vi "RSZVB Set Display Results State.vi"(7 "Display Results (F: Off)":bool, 8 "error in (no error)":errorcluster {"code" format="%.0x"}, 9 "Result Type (0: Phase Delay/El Length)":i32(ring) items=["Phase Delay/El Length", "Min/Max/Peak-Peak", "Mean/Std Dev", "RMS", "Gain/Slope/Flatness", "Compression Point"], 10 "Channel (Trace) (1)":i32=1, 11 "VISA session":refnum<visa-resource-name>) -> (0 "error out":errorcluster {"code" format="%.0x"}, 3 "dup VISA session":refnum<visa-resource-name>)   [LabVIEW 2011]
doc: "This VI displays or hides the Phase Delay/El Length, Min/Max/Peak-Peak, Mean/Std Dev, RMS, Gain/Slope/Flatness or Compression Point results in the diagram area of trace no. <Chn>.\n\nRemote-control command(s):\nCALCulate<Chn>:STATistics:EPDelay[:STATe] <Boolean>\nCALCulate<Chn>:STATistics:MMPTpeak[:STATe] <Boolean>\nCALCulate<Chn>:STATistics:MSTDdev[:STATe] <Boolean>\nCALCulate<Chn>:STATistics:RMS[:STATe] <Boolean>\nCALCulate<Chn>:STATistics:SFLatness[:STATe] <Boolean>\nCALCulate<Chn>:STATistics:NLINear:COMP[:STATe] <Boolean>"
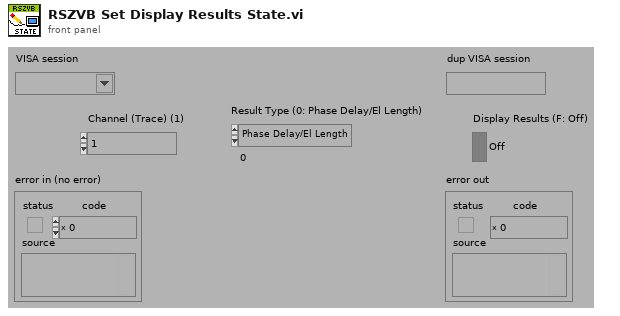
[diagram p1: front panel]
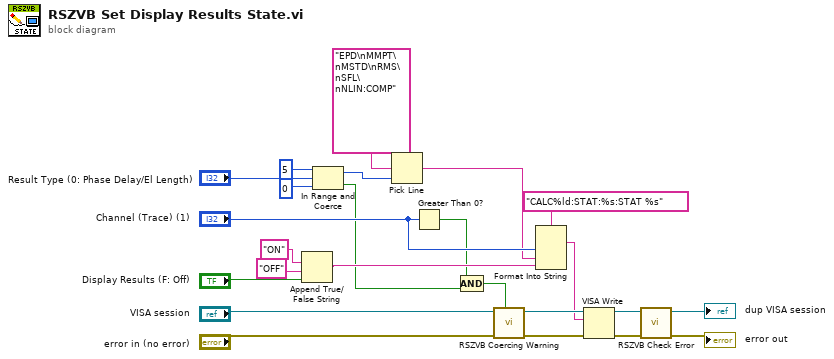
[diagram p0: block diagram]
diagram:
  n1 = Append True/False String(1:"Display Results (F: Off)", 2:"OFF", 3:"ON") -> (0:w9:string)  [unwired: 1 in]
  n2 = In Range and Coerce(upper limit=5 ("lower limit"), x="Result Type (0: Phase Delay/El Length)", lower limit=0) -> (coerced(x)=w5:i32, In Range?=w2:bool)
  n3 = Pick Line(multi-line string="EPD\nMMPT\nMSTD\nRMS\nSFL\nNLIN:COMP", line index=w5) -> (output string=w8:string)  [unwired: 1 in]
  n4 = Greater Than 0?(x="Channel (Trace) (1)") -> (x > 0?=w3:bool)
  n5 = Compound Arithmetic op=AND(w3, w2) -> (w1:bool)
  n6 = call "RSZVB Coercing Warning.vi"("In Range?"=w1, "error in (no error)"="error in (no error)", "VISA session"="VISA session") -> ("error out"=w21:errorcluster, "dup VISA session"=w22:refnum<visa-resource-name>)  [unwired: 7 in]
  n7 = Format Into String(format string="CALC%ld:STAT:%s:STAT %s", "Channel (Trace) (1)", w8, w9) -> (resulting string=w18:string)  [unwired: 2 in, 1 out]
  n8 = VISA Write(VISA resource name=w22, write buffer=w18, error in (no error)=w21) -> (VISA resource name out=w19:refnum<visa-resource-name>, error out=w20:errorcluster)  [unwired: 1 out]
  n9 = call "RSZVB Check Error.vi"("error in (no error)"=w20, "VISA session"=w19) -> ("error out"=→"error out":errorcluster, "dup VISA session"=→"dup VISA session":refnum<visa-resource-name>)  [unwired: 8 in]
